vi "Uninit.vi"(11 "DAQ DI in":refnum<class "DAQ DI.lvclass">) -> (3 "DAQ DI out":refnum<class "DAQ DI.lvclass">)   [LabVIEW 2020, in "DAQ DI.lvlib" / "DAQ DI.lvclass"]
doc: "This method is the inverse of the Pre Launch Init.vi. This method is called unconditionally at the end of an actor's lifetime, even if there was an error in Pre Launch Init.vi. Note that the self Enqueuer for the actor is already invalid by the time this VI executes: within this method, the actor may send messages to its caller but not to itself. This method executes before Last Ack is sent.\n\nThis method neither receives nor produces an error cluster. It is designed to provide an unconditional release of acquired resources. Any error raised during release is considered to be irrelevant to the actor's lifetime. If the actor truly needs to report some error status, it may send a message to caller or include information within itself that callers can examine when handling Last Ack."
uses:
  DAQ DI.lvclass
  DAQ DI.lvclass/DAQ DI.ctl
  <vilib>/ActorFramework/Actor/Actor.lvclass
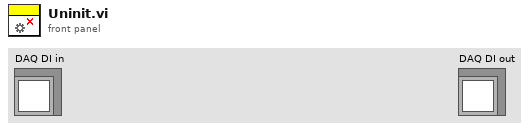
[diagram p1: front panel]
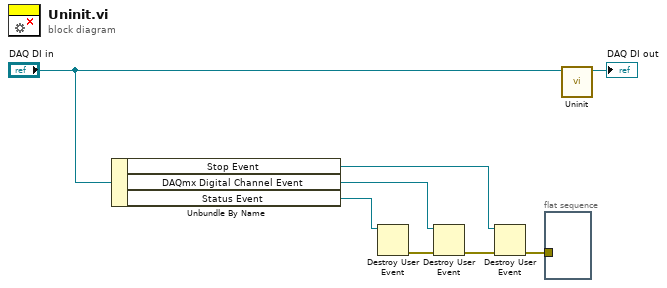
[diagram p0: block diagram]
diagram:
  n1 = Unbundle By Name("DAQ DI in") -> ("Stop Event"=w3:refnum<user-event>, "DAQmx Digital Channel Event"=w6:refnum<user-event>, "Status Event"=w7:refnum<user-event>)
  n2 = Destroy User Event(user event=w7) -> (error out=w5:errorcluster)  [unwired: 1 in]
  n3 = Destroy User Event(user event=w6, error in=w5) -> (error out=w4:errorcluster)
  n4 = Destroy User Event(user event=w3, error in=w4) -> (error out=w2:errorcluster)
  n5 = flat-sequence {
    tunnel: w2 -> [_]
    frame #0 {
    }
  }
  n6 = call-parent "Uninit.vi"("Actor in"="DAQ DI in") -> ("Actor out"=→"DAQ DI out":refnum<class "DAQ DI.lvclass">)  [unwired: 10 in]
